vi "WPI_RobotDriveArcadeDrive_StandardCUSTOM.vi"(6 "Wheel Difference":dbl, 8 "error in (no error)":errorcluster, 9 "Y axis value":dbl, 10 "X axis value":dbl, 11 "RobotDriveDevRef":T1={"DevStatus"={"status"=FALSE, "code"=0, "source"=""}, "Motors[]"=[], "Square Inputs"=FALSE, "Max Output"=1.0}) -> (0 "error out":errorcluster, 2 "Motor Values":dbl[](array[numeric]), 3 "RobotDriveDevRef":T1={"DevStatus"={"status"=FALSE, "code"=0, "source"=""}, "Motors[]"=[], "Square Inputs"=FALSE, "Max Output"=1.0})   [LabVIEW 2014]
doc: "Uses a standard algorithm to configure the motors for arcade driving. This algorithm does not saturate over half of the range.\n\nThis software is licensed. Open the labview\\readme\\WPI Robotics Library Open Source License.txt file for more information."
uses:
  <vilib>/Rock Robotics/WPI/RobotDrive/WPI_RobotDriveDevRef.ctl
  <vilib>/Rock Robotics/WPI/MotorControl/WPI_MotorControlDeviceRef.ctl
  <vilib>/Rock Robotics/WPI/MotorControl/WPI_MotorControlType.ctl
  <vilib>/Rock Robotics/SystemInterfaces/Typedef/FPGA_TypedefDigitalModule.ctl
  <vilib>/Rock Robotics/SystemInterfaces/DIO/FPGA_DIOPWMChannel.ctl
  <vilib>/Rock Robotics/WPI/PWM/WPI_PWMDeadband.ctl
  <vilib>/Rock Robotics/WPI/CAN/Jaguar/SubVIs/WPI_CANJaguar_ControlMode.ctl
  <vilib>/Rock Robotics/WPI/CAN/TalonSRX/WPI_CANTalonSRX_APIControlMode.ctl
  <vilib>/Rock Robotics/WPI/PWM/WPI_PWMTransform_ConPane.ctl
  <vilib>/Rock Robotics/WPI/RobotDrive/WPI_RobotDriveMotorSelectorEnum.ctl
  <vilib>/Rock Robotics/SystemInterfaces/NetworkCommunication/NetComm_UsageReport_ResourceType.ctl
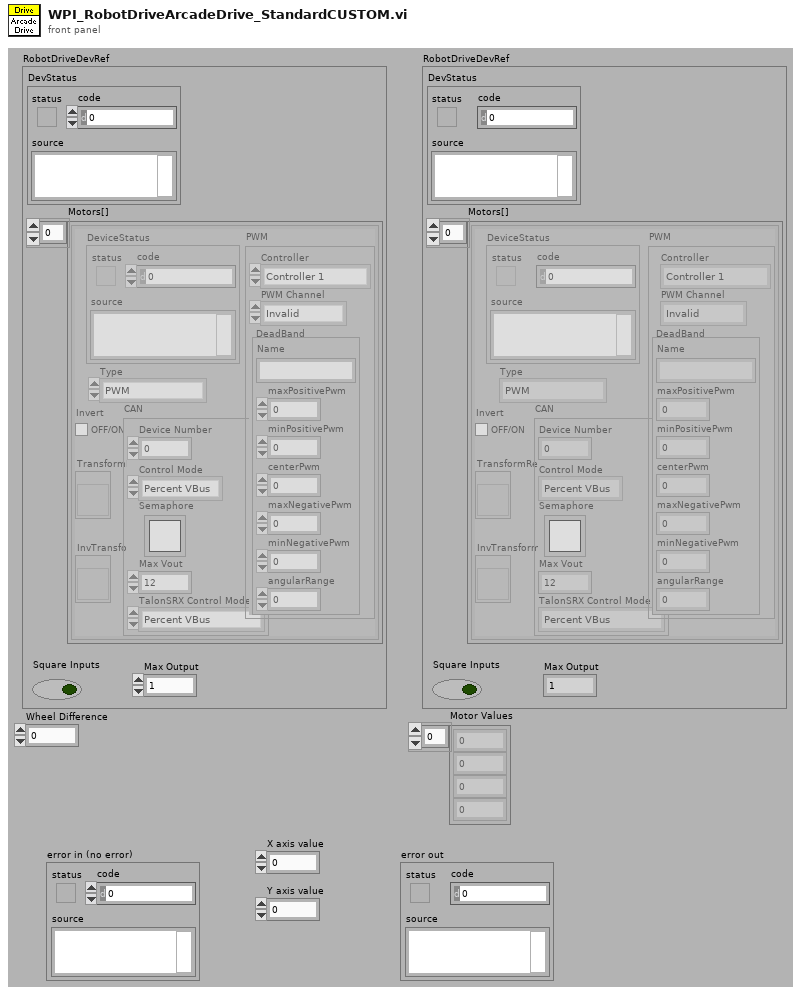
[diagram p1: front panel]
types:
  T1 = typedef "WPI_RobotDriveDevRef.ctl" = cluster{"DevStatus":errorcluster, "Motors[]":T2[], "Square Inputs":bool, "Max Output":dbl}
  T2 = typedef "WPI_MotorControlDeviceRef.ctl" = cluster{"DeviceStatus":errorcluster, "Type":T3, "PWM":cluster{"Controller":T4, "PWM Channel":T5, "DeadBand":T6}, "CAN":cluster{"Device Number":u8, "Control Mode":T7, "Semaphore":T8, "Max Vout":dbl, "TalonSRX Control Mode":T9}, "Invert":bool, "TransformRef":T10, "InvTransformRef":T10}
  T3 = typedef "WPI_MotorControlType.ctl" = enum16{"PWM", "CAN", "CANTalonSRX"}
  T4 = typedef "FPGA_TypedefDigitalModule.ctl" = enum16{"Controller 1"}
  T5 = typedef "FPGA_DIOPWMChannel.ctl" = enum8{"PWM 0", "PWM 1", "PWM 2", "PWM 3", "PWM 4", "PWM 5", "PWM 6", "PWM 7", "PWM 8", "PWM 9", "PWM MXP 0", "PWM MXP 1", "PWM MXP 2", "PWM MXP 3", "PWM MXP 4", "PWM MXP 5", "PWM MXP 6", "PWM MXP 7", "PWM MXP 8", "PWM MXP 9", "Invalid"}
  T6 = typedef "WPI_PWMDeadband.ctl" = cluster{"Name":string, "maxPositivePwm":i32, "minPositivePwm":i32, "centerPwm":i32, "maxNegativePwm":i32, "minNegativePwm":i32, "angularRange":u16}
  T7 = typedef "WPI_CANJaguar_ControlMode.ctl" = enum8{"Percent VBus", "Current", "Speed", "Position", "Voltage"}
  T8 = typedef "Semaphore RefNum" = refnum<k1>
  T9 = typedef "WPI_CANTalonSRX_APIControlMode.ctl" = enum8{"Percent VBus", "Speed", "Position", "Slave", "Unchanged / Invalid"}
  T10 = typedef "WPI_PWMTransform_ConPane.ctl" = refnum<vi>
  T11 = typedef "WPI_RobotDriveMotorSelectorEnum.ctl" = enum16{"Rear Left Motor", "Rear Right Motor", "Front Left Motor", "Front Right Motor"}
  T12 = typedef "NetComm_UsageReport_ResourceType.ctl" = enum8{"Controller", "Module", "Language", "CANPlugin", "Accelerometer", "ADXL345", "AnalogChannel", "AnalogTrigger", "AnalogTriggerOutput", "CANJaguar", "Compressor", "Counter", "Dashboard", "DigitalInput", "DigitalOutput", "DriverStationCIO", "DriverStationEIO", "DriverStationLCD", "Encoder", "GearTooth", "Gyro", "I2C", "Framework", "Jaguar", "Joystick", "Kinect", "KinectStick", "PIDController", "Preferences", "PWM", "Relay", "RobotDrive", "SerialPort", "Servo", "Solenoid", "SPI", "Task", "Ultrasonic", "Victor", "Button", "Command", "AxisCamera", "PCVideoServer", "SmartDashboard", "Talon", "HiTechnicColorSensor", "HiTechnicAccel", "HiTechnicCompass", "SRF08", "AnalogOutput", "Victor SP", "Talon SRX", "CAN Talon SRX"}
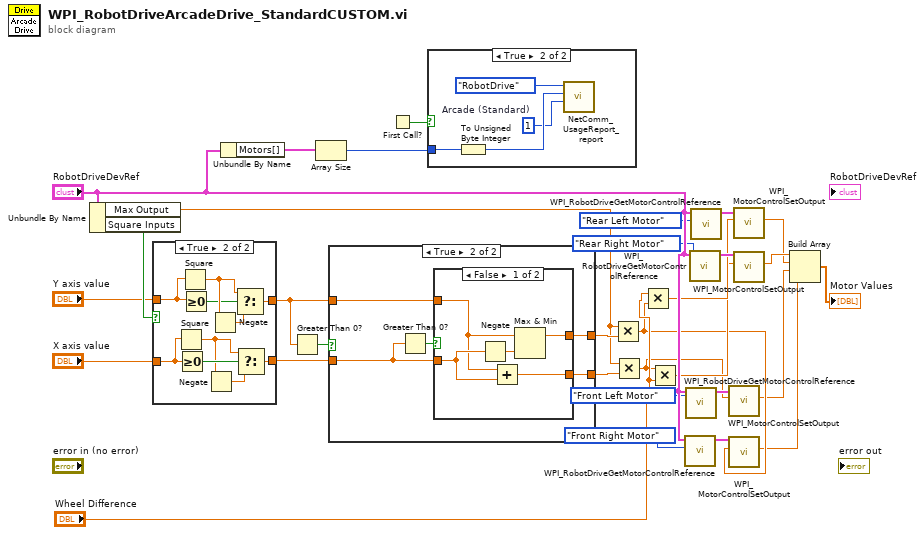
[diagram p0: block diagram]
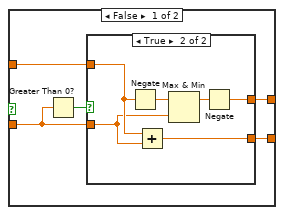
[diagram p3: hidden frame]
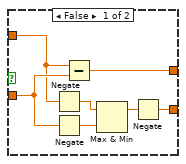
[diagram p4: hidden frame]
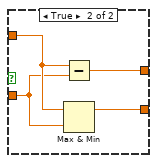
[diagram p5: hidden frame]
diagram:
  n1 = Unbundle By Name("RobotDriveDevRef") -> ("Max Output"=w23:dbl, "Square Inputs"=w31:bool)
  n2 = case shown="True" w31 {
    tunnel: [w32 w43] -> w28
    tunnel: [w33 w42] -> w29
    tunnel: "X axis value" -> [w32 w41]
    tunnel: "Y axis value" -> [w33 w40]
    frame False {
    }
    frame True {
      n3 = Square(x=w41) -> (x^2=w38:dbl)
      n4 = Greater Or Equal To 0?(x=w41) -> (x >= 0?=w39:bool)
      n5 = Square(x=w40) -> (x^2=w35:dbl)
      n6 = Greater Or Equal To 0?(x=w40) -> (x >= 0?=w34:bool)
      n7 = Negate(x=w38) -> (-x=w37:dbl)
      n8 = Negate(x=w35) -> (-x=w36:dbl)
      n9 = Select(t=w35, s=w34, f=w36) -> (s? t:f=w42:dbl)
      n10 = Select(t=w38, s=w39, f=w37) -> (s? t:f=w43:dbl)
    }
  }
  n11 = Unbundle By Name("RobotDriveDevRef") -> ("Motors[]"=w21:T2[])
  n12 = Greater Than 0?(x=w29) -> (x > 0?=w30:bool)
  n13 = Array Size(array=w21) -> (size(s)=w20:i32)
  n14 = case shown="True" w30 {
    tunnel: w28 -> [w47 w65]
    tunnel: w29 -> [w46 w64]
    tunnel: [w45 w63] -> w27
    tunnel: [w44 w62] -> w24
    frame False {
      n15 = Greater Than 0?(x=w47) -> (x > 0?=w48:bool)
      n16 = case shown="True" w48 {
        tunnel: w47 -> [w55 w57]
        tunnel: w46 -> [w53 w58]
        tunnel: [w49 w59] -> w45
        tunnel: [w50 w56] -> w44
        frame False {
          n17 = Negate(x=w53) -> (-x=w54:dbl)
          n18 = Negate(x=w55) -> (-x=w52:dbl)
          n19 = Subtract(x=w53, y=w55) -> (x-y=w49:dbl)
          n20 = Max & Min(x=w54, y=w52) -> (max(x,y)=w51:dbl)  [unwired: 1 out]
          n21 = Negate(x=w51) -> (-x=w50:dbl)
        }
        frame True {
          n22 = Negate(x=w58) -> (-x=w61:dbl)
          n23 = Add(x=w58, y=w57) -> (x+y=w56:dbl)
          n24 = Max & Min(x=w61, y=w57) -> (max(x,y)=w60:dbl)  [unwired: 1 out]
          n25 = Negate(x=w60) -> (-x=w59:dbl)
        }
      }
    }
    frame True {
      n26 = Greater Than 0?(x=w65) -> (x > 0?=w66:bool)
      n27 = case shown="False" w66 {
        tunnel: w65 -> [w71 w73]
        tunnel: w64 -> [w68 w74]
        tunnel: [w69 w72] -> w63
        tunnel: [w67 w75] -> w62
        frame False {
          n28 = Negate(x=w71) -> (-x=w70:dbl)
          n29 = Add(x=w68, y=w71) -> (x+y=w67:dbl)
          n30 = Max & Min(x=w68, y=w70) -> (max(x,y)=w69:dbl)  [unwired: 1 out]
        }
        frame True {
          n31 = Subtract(x=w74, y=w73) -> (x-y=w72:dbl)
          n32 = Max & Min(x=w74, y=w73) -> (max(x,y)=w75:dbl)  [unwired: 1 out]
        }
      }
    }
  }
  n33 = First Call?() -> (First Call?: T/F=w22:bool)
  n34 = case shown="True" w22 {
    tunnel: w20 -> [_ w78]
    frame False {
    }
    frame True {
      w76 = u8 1  # Arcade (Standard)
      n35 = To Unsigned Byte Integer(number=w78) -> (unsigned 8bit integer=w77:u8)
      n36 = call <vilib>:"NetComm_UsageReport_report.vi"("Context"=w76, "Instance Number"=w77, "Resource Type"=NetComm_UsageReport_ResourceType."RobotDrive") -> ()  [unwired: 9 in]
    }
  }
  n37 = Multiply(x=w23, y=w27) -> (x*y=w6:dbl)
  n38 = Multiply(x=w23, y=w24) -> (x*y=w7:dbl)
  n39 = Multiply(x="Wheel Difference", y=w6) -> (x*y=w9:dbl)
  n40 = Multiply(x=w7, y="Wheel Difference") -> (x*y=w8:dbl)
  n41 = call <vilib>:"WPI_RobotDriveGetMotorControlReference.vi"("MotorIndex"=WPI_RobotDriveMotorSelectorEnum."Front Right Motor", "RobotDriveDevRef"="RobotDriveDevRef") -> ("MotorControlDeviceRef"=w10:T2)  [unwired: 9 out]
  n42 = call <vilib>:"WPI_RobotDriveGetMotorControlReference.vi"("MotorIndex"=WPI_RobotDriveMotorSelectorEnum."Front Left Motor", "RobotDriveDevRef"="RobotDriveDevRef") -> ("MotorControlDeviceRef"=w11:T2)  [unwired: 9 out]
  n43 = call <vilib>:"WPI_RobotDriveGetMotorControlReference.vi"("MotorIndex"=WPI_RobotDriveMotorSelectorEnum."Rear Right Motor", "RobotDriveDevRef"="RobotDriveDevRef") -> ("MotorControlDeviceRef"=w12:T2)  [unwired: 9 out]
  n44 = call <vilib>:"WPI_RobotDriveGetMotorControlReference.vi"("MotorIndex"=WPI_RobotDriveMotorSelectorEnum."Rear Left Motor", "RobotDriveDevRef"="RobotDriveDevRef") -> ("MotorControlDeviceRef"=w13:T2)  [unwired: 9 out]
  n45 = call <vilib>:"WPI_MotorControlSetOutput.vi"("Output"=w7, "MotorControlDevRef"=w11) -> ("Motor Output"=w3:dbl)  [unwired: 7 in, 2 out]
  n46 = call <vilib>:"WPI_MotorControlSetOutput.vi"("Output"=w6, "MotorControlDevRef"=w10) -> ("Motor Output"=w2:dbl)  [unwired: 7 in, 2 out]
  n47 = call <vilib>:"WPI_MotorControlSetOutput.vi"("Output"=w9, "MotorControlDevRef"=w13) -> ("Motor Output"=w4:dbl)  [unwired: 7 in, 2 out]
  n48 = call <vilib>:"WPI_MotorControlSetOutput.vi"("Output"=w8, "MotorControlDevRef"=w12) -> ("Motor Output"=w5:dbl)  [unwired: 7 in, 2 out]
  n49 = Build Array(w5, w4, w3, w2) -> (→"Motor Values":dbl[])
